vi "로그인만들기.vi"() -> ()   [LabVIEW 2014]
panel:
  out "error in (no error) 2":errorcluster caption="error in (no error)"
  out "배열":string[](array[string])
  out "로그인?":bool
  in  "파일(대화 상자 사용)":path
  in  "error in (no error)":errorcluster caption="에러 입력(에러 없음)"
  in  "pw":string
  in  "id":string
  in  "취소 버튼":bool
  in  "확인 버튼":bool
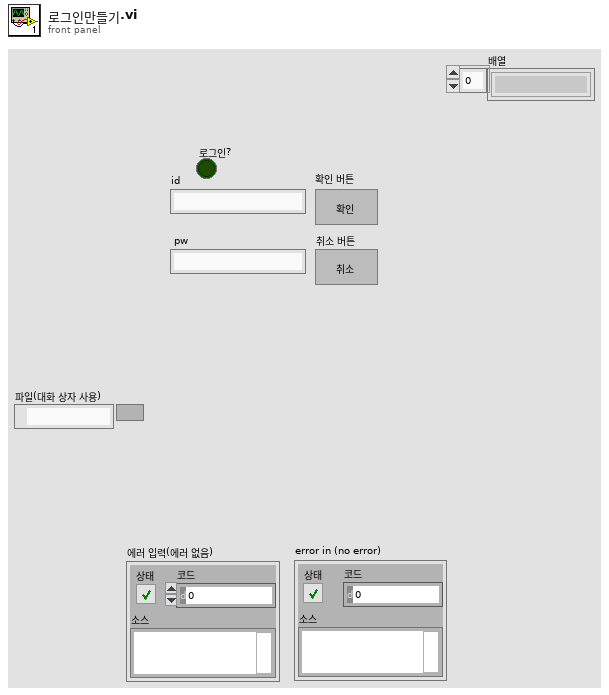
[diagram p1: front panel]
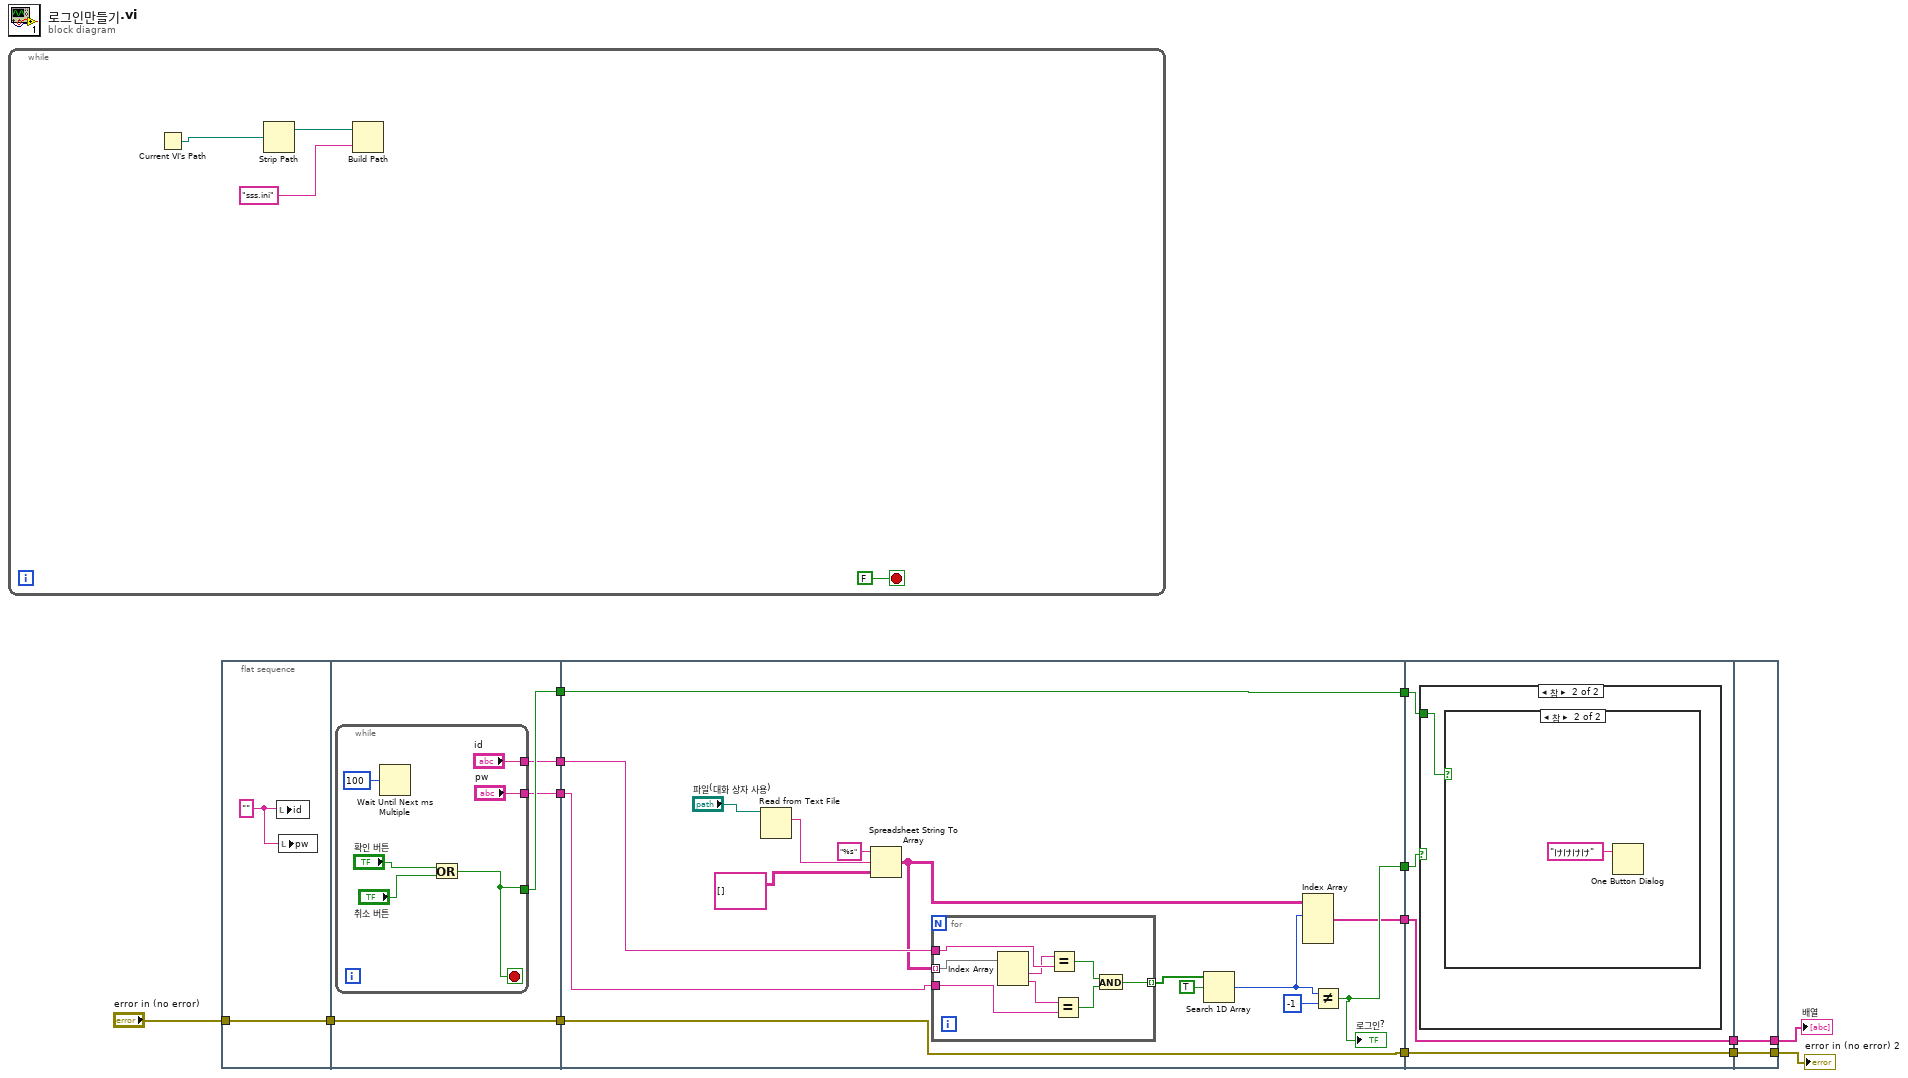
[diagram p0: block diagram]
diagram:
  n1 = while {
    stop <- FALSE stop-if-true
    n2 = Current VI's Path() -> (path=w17:path)
    n3 = Strip Path(path=w17) -> (stripped path=w16:path)  [unwired: 1 out]
    n4 = Build Path(base path=w16, name or relative path="sss.ini" ("이름 또는 상대 경로")) -> ()  [unwired: 1 out]
  }
  n5 = flat-sequence {
    tunnel: [w19] -> w11
    tunnel: "error in (no error)" -> [w19]
    tunnel: [w24] -> w14
    tunnel: [w23] -> w13
    tunnel: [w22] -> w12
    tunnel: w11 -> [w21]
    tunnel: [w21] -> w9
    tunnel: w14 -> [w45]
    tunnel: w13 -> [w39]
    tunnel: w12 -> [w40]
    tunnel: w9 -> [w32]
    tunnel: [w45] -> w8
    tunnel: [w33] -> w7
    tunnel: [w32] -> w6
    tunnel: [w31] -> w5
    tunnel: w8 -> [w56]
    tunnel: w7 -> [w57]
    tunnel: w6 -> [w55]
    tunnel: w5 -> [w54]
    tunnel: [w55] -> w4
    tunnel: [w54] -> w3
    tunnel: [w61] -> w2
    tunnel: [w62] -> w1
    tunnel: w4 -> [w62]
    tunnel: w3 -> [w61]
    frame #0 {
      w20 = ""
      n6 = local write "id"(w20) -> ()
      n7 = local write "pw"(w20) -> ()
    }
    frame #1 {
      n8 = while {
        tunnel: [w27] -> w24
        tunnel: ["pw"] -> w23
        tunnel: ["id"] -> w22
        stop <- w27 stop-if-true
        n9 = Wait Until Next ms Multiple(millisecond multiple=u32 100 ("ms 배수")) -> ()  [unwired: 1 out]
        n10 = Or(x="확인 버튼", y="취소 버튼") -> (x .or. y?=w27:bool)
      }
    }
    frame #2 {
      n11 = Read from Text File(file (use dialog)="파일(대화 상자 사용)") -> (text=w43:string)  [unwired: 3 in, 3 out]
      n12 = Spreadsheet String To Array(format string="%s" ("포맷 문자열"), spreadsheet string=w43, array type (2D Dbl)=string[][] []) -> (array=w38:string[][])  [unwired: 1 in]
      n13 = for {
        tunnel: w40 -> [w52]
        tunnel: w39 -> [w49]
        tunnel: w38 -> [w53] mode=indexing
        tunnel: [w46] -> w37 mode=indexing
        n14 = Index Array(array=w53) -> (element #1=w51:string, element #2=w50:string)  [unwired: 2 in]
        n15 = Equal?(x=w51, y=w52) -> (x = y?=w47:bool)
        n16 = Equal?(x=w50, y=w49) -> (x = y?=w48:bool)
        n17 = And(x=w47, y=w48) -> (x .and. y?=w46:bool)
      }
      n18 = Search 1D Array(1D array=w37, element=TRUE ("원소")) -> (index of element=w35:i32)  [unwired: 1 in]
      n19 = Index Array(array=w38, index (row) #1=w35) -> (element #1=w31:string[])  [unwired: 3 in, 1 out]
      n20 = Not Equal?(x=w35, y=-1) -> (x != y?=w33:bool)
      "로그인?" <- w33
    }
    frame #3 {
      n21 = case shown="참" w57 {
        tunnel: w56 -> [w58 w59]
        frame False {
          n22 = case shown="참" w58 {
            frame False {
            }
            frame True {
            }
          }
        }
        frame True {
          n23 = case shown="참" w59 {
            frame False {
            }
            frame True {
              n24 = One Button Dialog(message="けけけけ" ("메시지")) -> ()  [unwired: 1 in, 1 out]
            }
          }
        }
      }
    }
    frame #4 {
    }
  }
  "배열" <- w2
  "error in (no error) 2" <- w1
